vi "SensorLoopQCP.vi"   [LabVIEW 2017]
uses:
  <userlib>/836-Library/System/QCP_V2/QCPSupportCode/QCP_GetDbl.vi
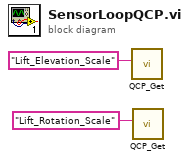
[diagram p0: block diagram]
diagram:
  n1 = call-poly <userlib>:"QCP_Get.vi"("Value Name"="Lift_Elevation_Scale") -> ()  [unwired: 8 in, 3 out]
  n2 = call-poly <userlib>:"QCP_Get.vi"("Value Name"="Lift_Rotation_Scale") -> ()  [unwired: 8 in, 3 out]
